vi "DSC Dashboard.vi"() -> ()   [LabVIEW 2016]
uses:
  OAuth/OO OAuth/scope_needed.ctl
  <vilib>/addons/_JKI.lib/REST Client/classes/REST Client/HTTP Header.ctl
  <vilib>/addons/_JKI.lib/REST Client/classes/REST Client/REST Client.lvclass
panel:
  out "Response body":string
  in  "Update Button":bool
  in  "OK":bool
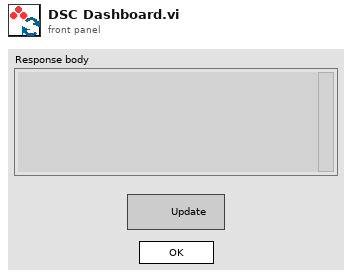
[diagram p1: front panel]
types:
  T1 = enum32{"Invalid", "Standard", "Closed", "Hidden", "Minimized", "Maximized"}
  T2 = enum32{"invalid app kind", "Development System", "Run Time System", "Student Edition", "Embedded LabVIEW", "Evaluation", "Custom"}
  T3 = cluster{"Client ID":string, "Client Secret":string, "Redirect URI":string, "Token Endpoint":string, "Scope":string}
  T4 = typedef "scope_needed.ctl" = enum16{"No", "Yes"}
  T5 = typedef "REST Client.lvlib/REST Client.lvclass/HTTP Header.ctl" = cluster{"header":string, "value":string}
  T6 = cluster{"Core":cluster{"Current VI Reference":refnum<vi>, "Close Panel on Exit?":bool}, "Access Token":string, "Auth Timeout":dbl, "Refresh Token":string, "DSC Data":cluster{"Cyper Temp":dbl, "PPMS1 Temp":dbl, "PPMS1 B-field":dbl, "PPMS2 Temp":dbl, "PPMS2 B-Field":dbl, "PPMS2 He Level":dbl, "THZ1 Temp":dbl, "THZ1 Humidity":dbl, "THZ1 Dew Pt":dbl}}
  T7 = cluster{"Cyper Temp":dbl, "PPMS1 Temp":dbl, "PPMS1 B-field":dbl, "PPMS2 Temp":dbl, "PPMS2 B-Field":dbl, "PPMS2 He Level":dbl, "THZ1 Temp":dbl, "THZ1 Humidity":dbl, "THZ1 Dew Pt":dbl}
  T8 = cluster{"Current VI Reference":refnum<vi>, "Close Panel on Exit?":bool}
  T9 = cluster{"Cypher Temp":dbl, "PPMS1 Temp":dbl, "PPMS1 B-Field":dbl, "PPMS2 Temp":dbl, "PPMS2 B-field":dbl, "PPMS2 He level":dbl, "THZ1 Temp":dbl, "THZ1 Humidity":dbl, "THZ1 Dew Pt":dbl}
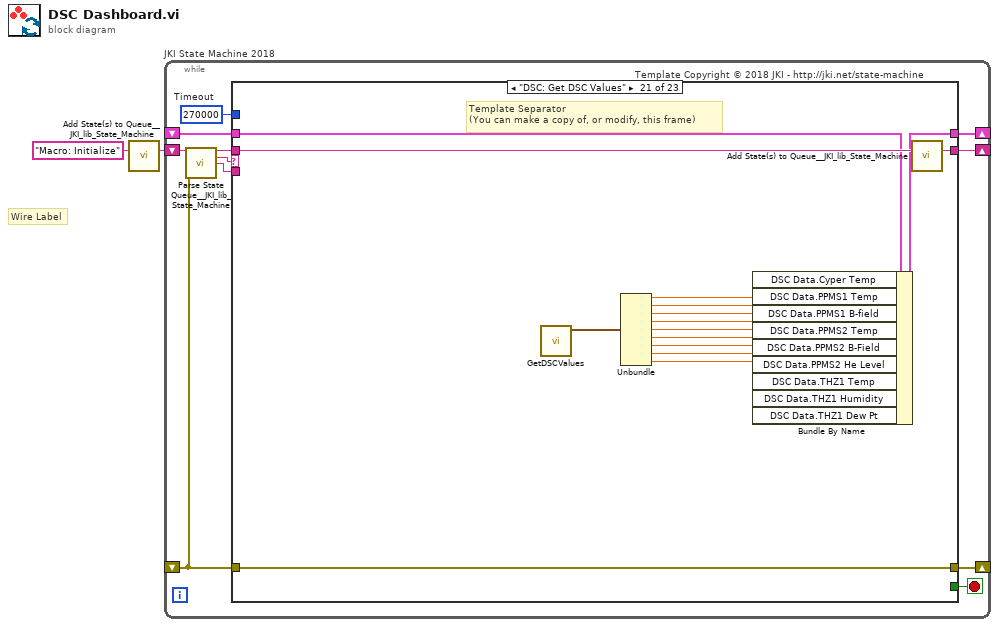
[diagram p0: block diagram]
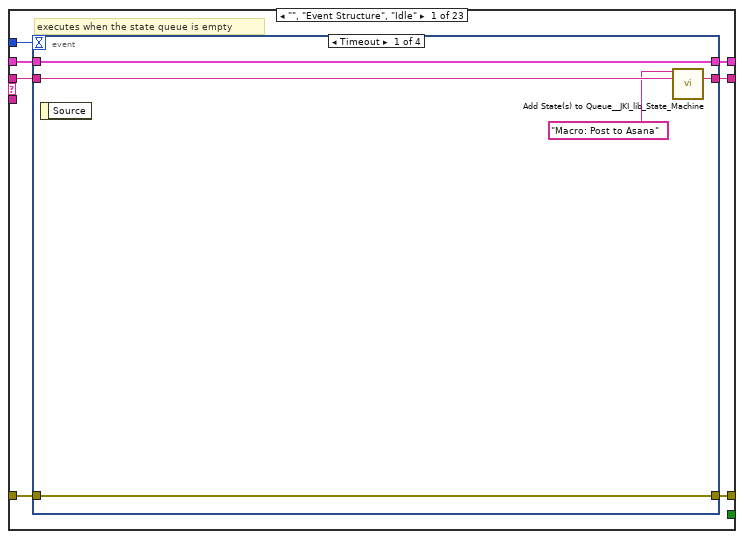
[diagram p2: hidden frame]
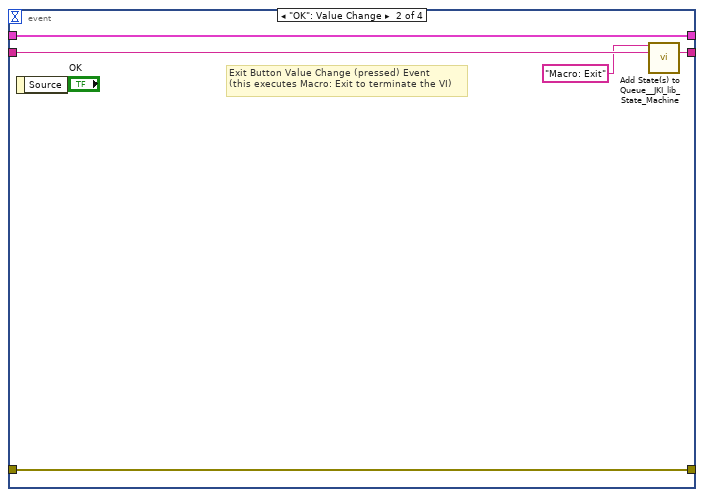
[diagram p3: hidden frame]
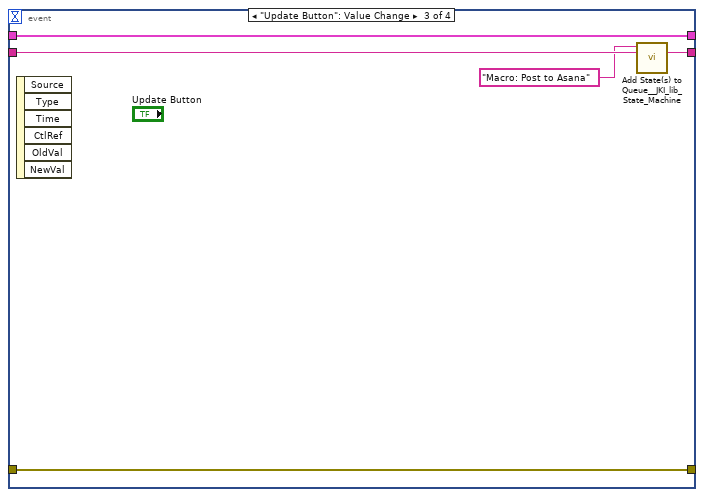
[diagram p4: hidden frame]
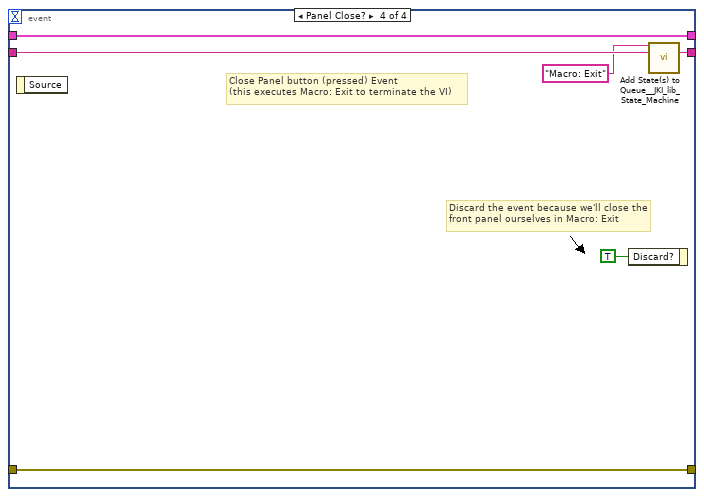
[diagram p5: hidden frame]
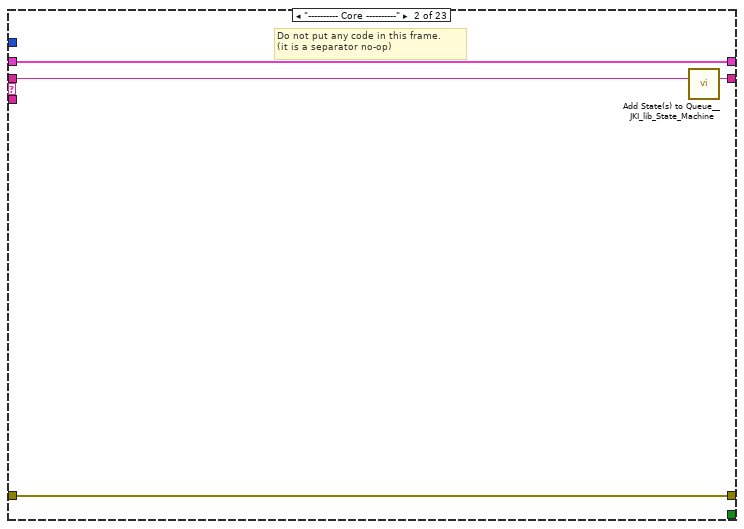
[diagram p6: hidden frame]
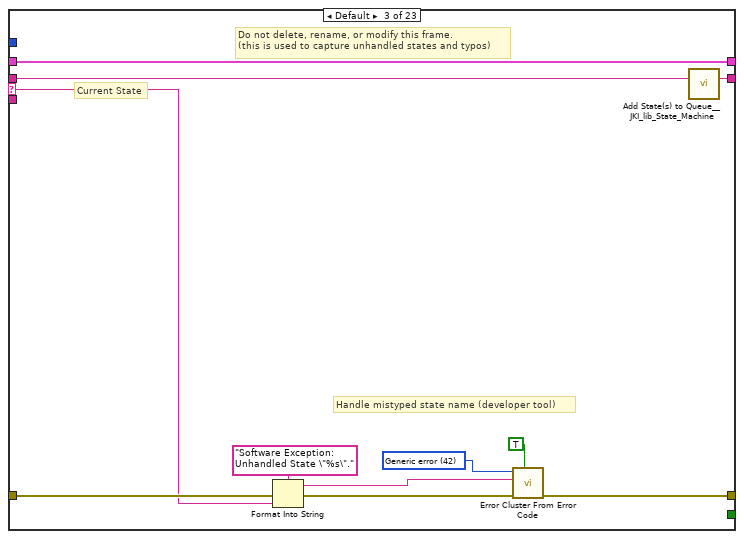
[diagram p7: hidden frame]
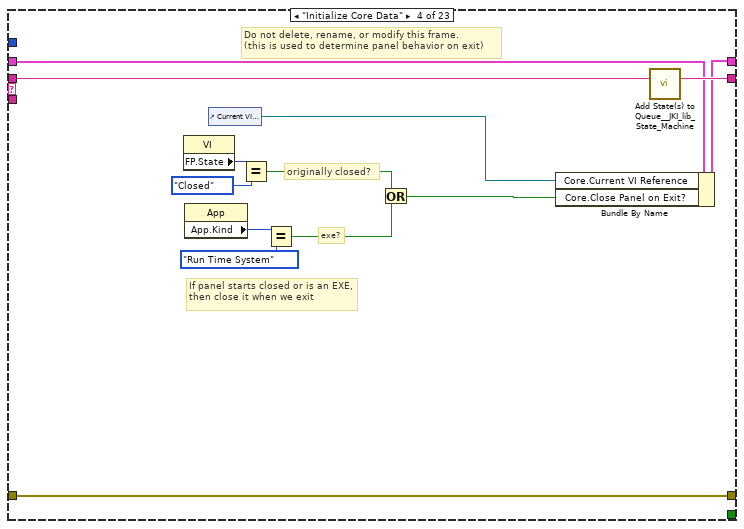
[diagram p8: hidden frame]
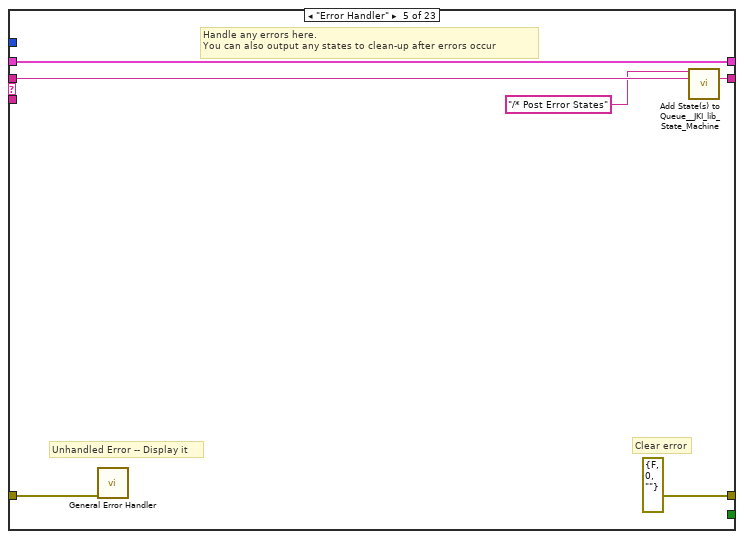
[diagram p9: hidden frame]
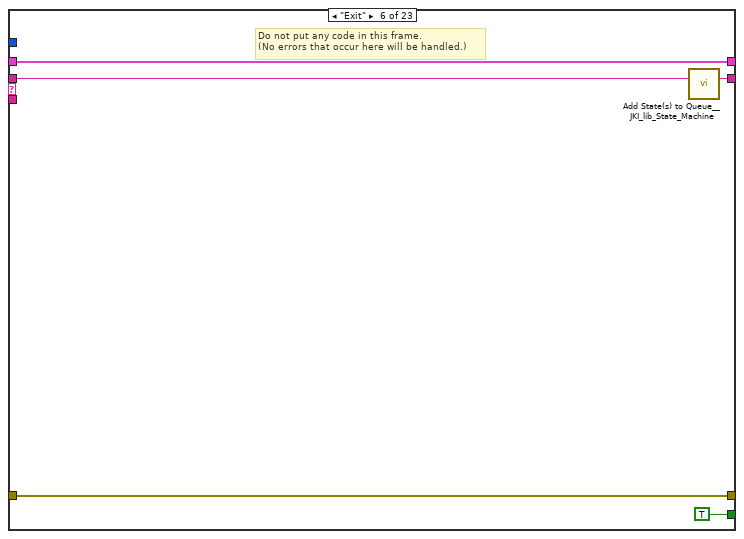
[diagram p10: hidden frame]
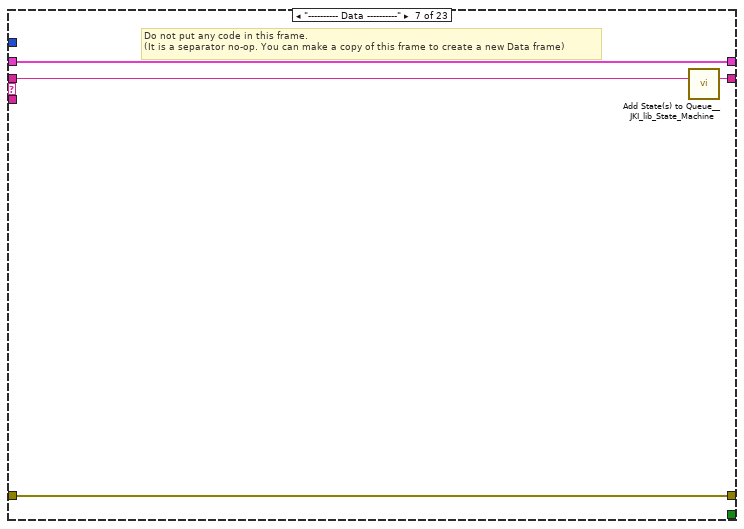
[diagram p11: hidden frame]
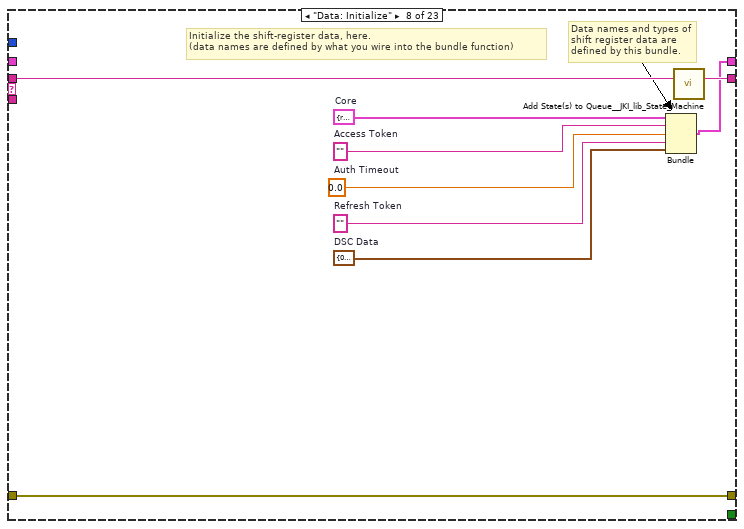
[diagram p12: hidden frame]
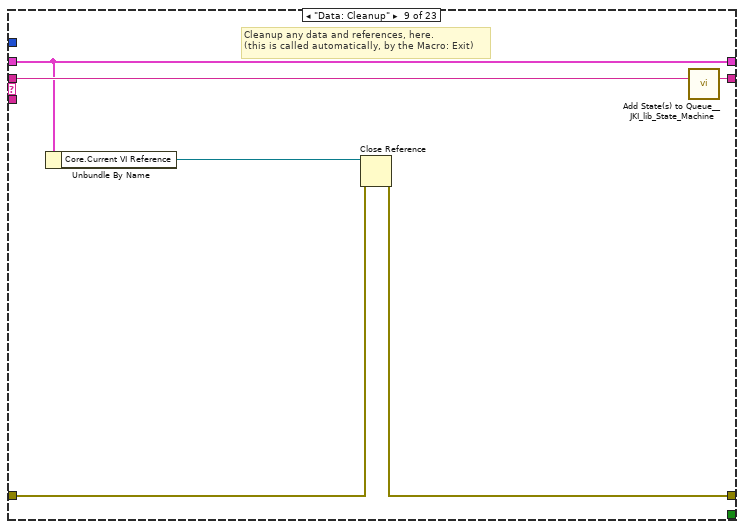
[diagram p13: hidden frame]
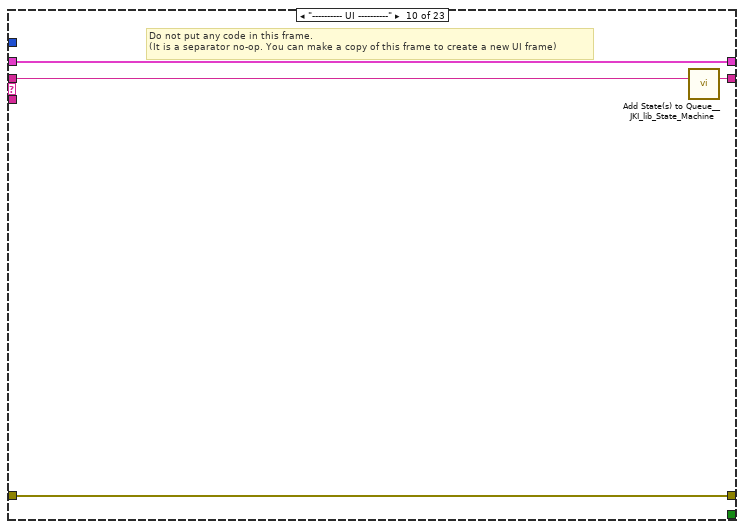
[diagram p14: hidden frame]
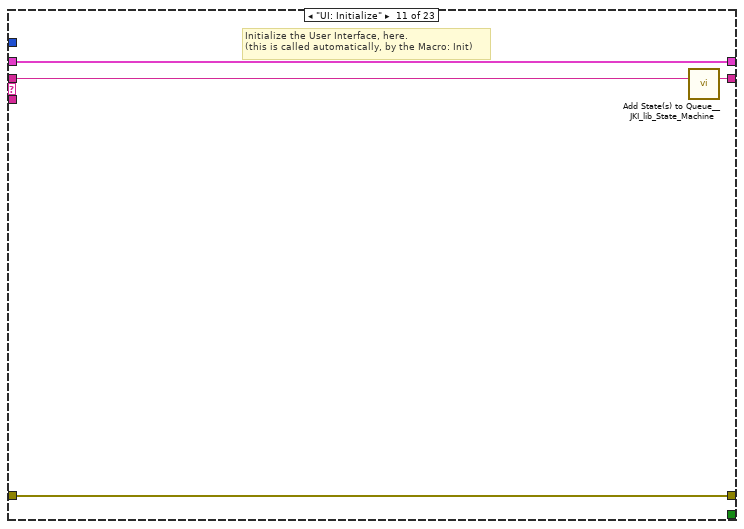
[diagram p15: hidden frame]
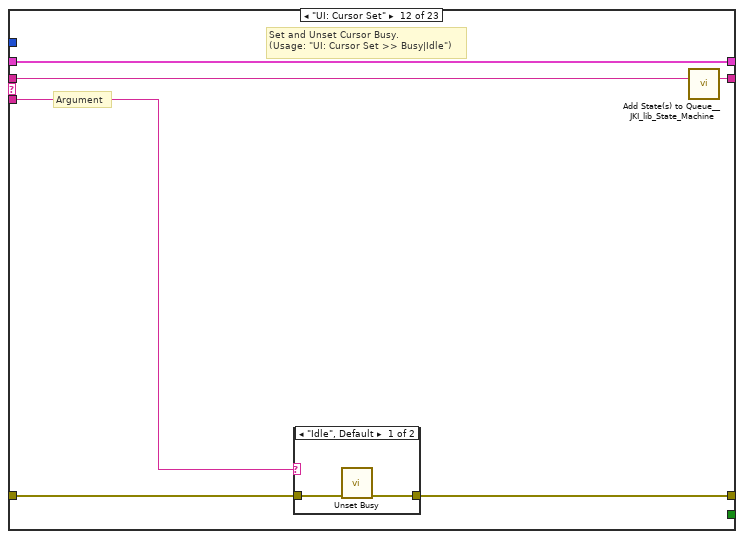
[diagram p16: hidden frame]
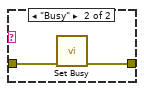
[diagram p17: hidden frame]
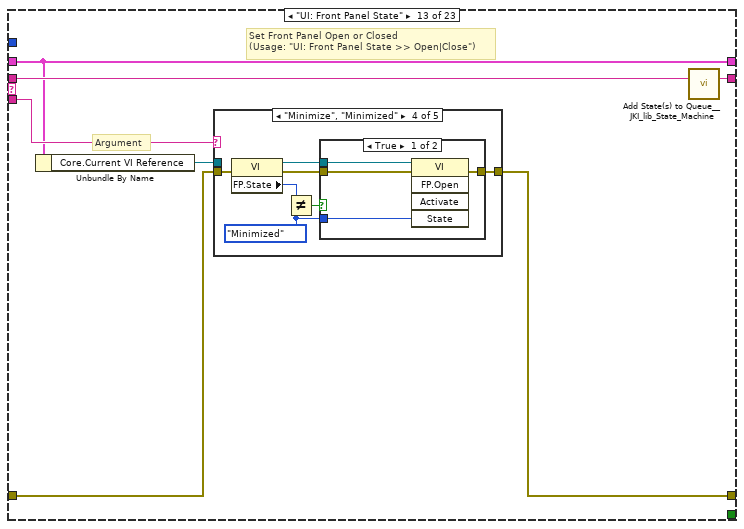
[diagram p18: hidden frame]
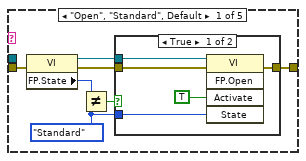
[diagram p19: hidden frame]
diagram:
  # "Wire Label"
  n1 = call <vilib>:"Add State(s) to Queue__JKI_lib_State_Machine.vi"("State(s) in (\"\")"="Macro: Initialize") -> ("States Out"=w2:string)  [unwired: 14 in]
  n2 = while "JKI State Machine 2018" {
    shift-right: [w3] -> _
    shift-left: _ -> [w6]
    shift-right: [w9] -> _
    shift-left: _ -> [w4]
    shift-right: [w8] -> _
    shift-left: w2 -> [w10]
    stop <- w7 stop-if-true
    w5 = 270000  # Timeout
    # "Template Copyright © 2018 JKI - http://jki.net/state-machine"
    n3 = call <vilib>:"Parse State Queue__JKI_lib_State_Machine.vi"("State Queue"=w10, "Error In (no error)"=w4) -> ("Remaining States"=w12:string, "Current State"=w13:string, "Arguments"=w11:string)  [unwired: 11 in]
    n4 = case shown="\"DSC: Get DSC Values\"" w13 {
      selector: w13 -> [_ _ w46 _ _ _ _ _ _ _ _ _ _ _ _ _ _ _ _ _ _ _ _]
      tunnel: w12 -> [w20 w45 w50 w69 w75 w80 w84 w93 w99 w103 w107 w113 w124 w188 w193 w198 w208 w212 w223 w239 w254 w258 w280]
      tunnel: w11 -> [_ _ _ _ _ _ _ _ _ _ _ w108 w119 _ _ _ _ _ _ _ _ _ _]
      tunnel: w6 -> [w18 w42 w48 w57 w72 w78 w81 _ w94 w100 w105 w111 w118 w185 w190 w195 w200 w209 w215 w236 w241 w255 w263]
      tunnel: [w17 w43 w52 w67 errorcluster {"status"=FALSE, "code"=0, "source"=""} ("error out") w77 w82 w91 w96 w101 w104 w109 w121 w186 w191 w196 w206 w210 w216 w237 w252 w256 w259] -> w9
      tunnel: w4 -> [w16 w43 w51 w67 w71 w77 w82 w91 w97 w101 w104 w110 w122 w186 w191 w196 w206 w210 w217 w237 w252 w256 w262]
      tunnel: [w19 w44 w49 w68 w74 w79 w83 w92 w98 w102 w106 w112 w123 w187 w192 w197 w207 w211 w222 w238 w253 w257 w279] -> w8
      tunnel: [_ _ _ _ _ TRUE _ _ _ _ _ _ _ _ _ _ _ _ _ _ _ _ _] -> w7
      tunnel: w5 -> [w14 _ _ _ _ _ _ _ _ _ _ _ _ _ _ _ _ _ _ _ _ _ _]
      tunnel: [w15 w42 w48 w58 w72 w78 w81 w88 w94 w100 w105 w111 w118 w185 w190 w195 w200 w209 w214 w236 w240 w255 w263] -> w3
      frame "", "Event Structure", "Idle" {
        # "executes when the state queue is empty"
        n5 = event shown="[0] Timeout" {
          selector: _ -> [_ _ _ _]
          dyn-events: _ -> [_ _ _ _]
          timeout: w14 -> [_ _ _ _]
          tunnel: w20 -> [w25 w30 w33 w41]
          tunnel: [w24 w29 w34 w40] -> w19
          tunnel: w18 -> [w22 w27 w35 w38]
          tunnel: [w23 w28 w31 w39] -> w17
          tunnel: w16 -> [w23 w28 w31 w39]
          tunnel: [w22 w27 w35 w38] -> w15
          event Timeout {
            n6 = event-data() -> ()  [unwired: 1 in, 1 out]
            n7 = call <vilib>:"Add State(s) to Queue__JKI_lib_State_Machine.vi"("State(s) in Front (\"\")"="Macro: Post to Asana" ("State(s) in Front (\"\")"), "State(s) in (\"\")"=w25) -> ("States Out"=w24:string)  [unwired: 13 in]
          }
          event "OK": Value Change {
            # "Exit Button Value Change (pressed) Event\n(this executes Macro: Exit to terminate the VI)"
            n8 = event-data() -> ()  [unwired: 1 in, 1 out]
            n9 = call <vilib>:"Add State(s) to Queue__JKI_lib_State_Machine.vi"("State(s) in Front (\"\")"="Macro: Exit", "State(s) in (\"\")"=w30) -> ("States Out"=w29:string)  [unwired: 13 in]
          }
          event "Update Button": Value Change {
            n10 = event-data() -> ()  [unwired: 1 in, 6 out]
            n11 = call <vilib>:"Add State(s) to Queue__JKI_lib_State_Machine.vi"("State(s) in Front (\"\")"="Macro: Post to Asana", "State(s) in (\"\")"=w33) -> ("States Out"=w34:string)  [unwired: 13 in]
          }
          event Panel Close? {
            # "Discard the event because we'll close the front panel ourselves in Macro: Exit"
            # "Close Panel button (pressed) Event\n(this executes Macro: Exit to terminate the VI)"
            n12 = event-data() -> ()  [unwired: 1 in, 1 out]
            n13 = event-data("Discard?"=TRUE) -> ()  [unwired: 1 in, 1 out]
            n14 = call <vilib>:"Add State(s) to Queue__JKI_lib_State_Machine.vi"("State(s) in Front (\"\")"="Macro: Exit", "State(s) in (\"\")"=w41) -> ("States Out"=w40:string)  [unwired: 13 in]
          }
        }
      }
      frame "---------- Core ----------" {
        # "Do not put any code in this frame.\n(it is a separator no-op)"
        n15 = call <vilib>:"Add State(s) to Queue__JKI_lib_State_Machine.vi"("State(s) in (\"\")"=w45) -> ("States Out"=w44:string)  [unwired: 14 in]
      }
      frame Default {
        w55 = 42 items=["No error", "Argument error", "Memory is full", "Out of zone", "End of file", "File already open", "Generic file I/O error", "File not found", "File permission error", "Disk is full", "Duplicate path", "Too many files open", "System feature not enabled", "Resource file not found", "Cannot add resource", "Resource not found", "Image not found", "Image memory error", "Pen does not exist", "Config type invalid", "Config token not found", "Config parse error", "Config memory error", "Bad external code format", "Bad external code offset", "External code not present", "Null window", "Destroy window error", "Null menu", "Print aborted", "Bad print record", "Print driver error", "Windows error during printing", "Memory error during printing", "Print dialog error", "Generic print error", "Invalid device refnum", "Device not found", "Device parameter error", "Device unit error", "Cannot open device", "Device call aborted", "Generic error", "Cancelled by user", "Object ID too low", "Object ID too high", "Object not in heap", "Unknown heap", "Unknown object (invalid DefProc)", "Unknown object (DefProc not in table)", "Message out of range", "Invalid (null) method", "Unknown message", "Manager call not supported", "Bad address", "Network operation in progress", "Network operation timed out", "Connection is busy", "Network attribute not supported", "Network error", "Address in use", "System out of memory", "Connection aborted", "Connection refused", "Not connected", "Already connected", "Connection closed", "Initialization error (interapplication manager)", "Bad occurrence", "Wait on unbound occurrence handler", "Occurrence queue overflow", "Datalog type conflict", "Unused", "Unrecognized type (interapplication manager)", "Memory corrupt", "Failed to make temporary DLL", "Old CIN version", "Drag socket not found", "Failed to load drop-object", "Failed to register OLE object", "Failed to release OLE object", "Format specifier type mismatch", "Unknown format specifier", "Too few format specifiers", "Too many format specifiers", "Scan failed", "Newer CIN version", "Error converting to variant", "Runtime menu error", "Password tampered", "Variant attribute not found", "Incompatible variant data type", "Event data is not available", "Event Store is not present", "Occurrence is not found", "Event Queue is not created", "Event info is not available", "Refnum passed is NULL", "Error retrieving Class GUID", "Error retrieving CoClass GUID", "Error retrieving TypeLib GUID.", "Bad built application magic bytes.", "Specific driver is different from the specific driver associated with the Logical Name.", "There is no session opened to the class driver.", "Max Error", "MAX - Error with config objects", "MAX - Error loading configuration", "MAX - Group not supported"]
        # "Current State"
        # "Do not delete, rename, or modify this frame.\n(this is used to capture unhandled states and typos)"
        # "Handle mistyped state name (developer tool)"
        n16 = Format Into String(format string="Software Exception: Unhandled State \"%s\"." ("message"), error in=w51, w46) -> (resulting string=w54:string, error out=w53:errorcluster)  [unwired: 1 in]
        n17 = call <vilib>:"Error Cluster From Error Code.vi"("show call chain? (False)"=TRUE, "error in (no error)"=w53, "error message (\"\")"=w54, "error code (0)"=w55) -> ("error out"=w52:errorcluster)  [unwired: 5 in]
        n18 = call <vilib>:"Add State(s) to Queue__JKI_lib_State_Machine.vi"("State(s) in (\"\")"=w50) -> ("States Out"=w49:string)  [unwired: 14 in]
      }
      frame "Initialize Core Data" {
        # "Do not delete, rename, or modify this frame.\n(this is used to determine panel behavior on exit)"
        # "originally closed?"
        # "exe?"
        # "If panel starts closed or is an EXE, then close it when we exit"
        n19 = property class="VI"() -> ("FP.State"=w61:T1)  [unwired: 2 in, 2 out]
        n20 = property class="App"() -> ("App.Kind"=w66:T2)  [unwired: 2 in, 2 out]
        n21 = control-ref of="Current VI Reference"() -> (w62:refnum<vi>)
        n22 = Equal?(x=w61, y=T1."Closed" ("Front Panel Window:State")) -> (x = y?=w59:bool)
        n23 = Equal?(x=w66, y=T2."Run Time System" ("Application:Kind")) -> (x = y?=w64:bool)
        n24 = Or(x=w59, y=w64) -> (x .or. y?=w63:bool)
        n25 = Bundle By Name(cluster=w57, "Core.Current VI Reference"=w62, "Core.Close Panel on Exit?"=w63) -> (w58:T6)
        n26 = call <vilib>:"Add State(s) to Queue__JKI_lib_State_Machine.vi"("State(s) in (\"\")"=w69) -> ("States Out"=w68:string)  [unwired: 14 in]
      }
      frame "Error Handler" {
        # "Unhandled Error -- Display it"
        # "Handle any errors here.\nYou can also output any states to clean-up after errors occur"
        # "Clear error"
        n27 = call <vilib>:"General Error Handler.vi"("error in (no error)"=w71) -> ()  [unwired: 10 in, 5 out]
        n28 = call <vilib>:"Add State(s) to Queue__JKI_lib_State_Machine.vi"("State(s) in Front (\"\")"="/* Post Error States", "State(s) in (\"\")"=w75) -> ("States Out"=w74:string)  [unwired: 13 in]
      }
      frame "Exit" {
        # "Do not put any code in this frame.\n(No errors that occur here will be handled.)"
        n29 = call <vilib>:"Add State(s) to Queue__JKI_lib_State_Machine.vi"("State(s) in (\"\")"=w80) -> ("States Out"=w79:string)  [unwired: 14 in]
      }
      frame "---------- Data ----------" {
        # "Do not put any code in this frame.\n(It is a separator no-op. You can make a copy of this frame to create a new Data frame)"
        n30 = call <vilib>:"Add State(s) to Queue__JKI_lib_State_Machine.vi"("State(s) in (\"\")"=w84) -> ("States Out"=w83:string)  [unwired: 14 in]
      }
      frame "Data: Initialize" {
        w85 = T7 {"Cyper Temp"=0.0, "PPMS1 Temp"=0.0, "PPMS1 B-field"=0.0, "PPMS2 Temp"=0.0, "PPMS2 B-Field"=0.0, "PPMS2 He Level"=0.0, "THZ1 Temp"=0.0, "THZ1 Humidity"=0.0, "THZ1 Dew Pt"=0.0}  # DSC Data
        w86 = ""  # Refresh Token
        w87 = ""  # Access Token
        w89 = 0.0  # Auth Timeout
        w90 = T8 {"Current VI Reference"=refnum, "Close Panel on Exit?"=FALSE}  # Core
        # "Data names and types of shift register data are defined by this bundle."
        # "Initialize the shift-register data, here.\n(data names are defined by what you wire into the bundle function)"
        n31 = Bundle("Core"=w90, "Access Token"=w87, "Auth Timeout"=w89, "Refresh Token"=w86, "DSC Data"=w85) -> (w88:T6)  [unwired: 1 in]
        n32 = call <vilib>:"Add State(s) to Queue__JKI_lib_State_Machine.vi"("State(s) in (\"\")"=w93) -> ("States Out"=w92:string)  [unwired: 14 in]
      }
      frame "Data: Cleanup" {
        # "Cleanup any data and references, here.\n(this is called automatically, by the Macro: Exit)"
        n33 = Unbundle By Name(w94) -> ("Core.Current VI Reference"=w95:refnum<vi>)
        n34 = Close Reference(reference=w95, error in (no error)=w97) -> (error out=w96:errorcluster)
        n35 = call <vilib>:"Add State(s) to Queue__JKI_lib_State_Machine.vi"("State(s) in (\"\")"=w99) -> ("States Out"=w98:string)  [unwired: 14 in]
      }
      frame "---------- UI ----------" {
        # "Do not put any code in this frame.\n(It is a separator no-op. You can make a copy of this frame to create a new UI frame)"
        n36 = call <vilib>:"Add State(s) to Queue__JKI_lib_State_Machine.vi"("State(s) in (\"\")"=w103) -> ("States Out"=w102:string)  [unwired: 14 in]
      }
      frame "UI: Initialize" {
        # "Initialize the User Interface, here.\n(this is called automatically, by the Macro: Init)"
        n37 = call <vilib>:"Add State(s) to Queue__JKI_lib_State_Machine.vi"("State(s) in (\"\")"=w107) -> ("States Out"=w106:string)  [unwired: 14 in]
      }
      frame "UI: Cursor Set" {
        # "Argument"
        # "Set and Unset Cursor Busy.\n(Usage: \"UI: Cursor Set >> Busy|Idle\")"
        n38 = case shown="\"Idle\", Default" w108 {
          tunnel: w110 -> [w115 w117]
          tunnel: [w114 w116] -> w109
          frame "Idle", Default {
            n39 = call <vilib>:"Unset Busy.vi"("error in (no error)"=w115) -> ("error out"=w114:errorcluster)  [unwired: 10 in]
          }
          frame "Busy" {
            n40 = call <vilib>:"Set Busy.vi"("error in (no error)"=w117) -> ("error out"=w116:errorcluster)  [unwired: 9 in, 1 out]
          }
        }
        n41 = call <vilib>:"Add State(s) to Queue__JKI_lib_State_Machine.vi"("State(s) in (\"\")"=w113) -> ("States Out"=w112:string)  [unwired: 14 in]
      }
      frame "UI: Front Panel State" {
        # "Argument"
        # "Set Front Panel Open or Closed\n(Usage: \"UI: Front Panel State >> Open|Close\")"
        n42 = Unbundle By Name(w118) -> ("Core.Current VI Reference"=w120:refnum<vi>)
        n43 = case shown="\"Minimize\", \"Minimized\"" w119 {
          tunnel: w122 -> [w130 w143 w154 w166 w178]
          tunnel: [w131 w144 w155 w167 w179] -> w121
          tunnel: w120 -> [_ _ _ _ _]
          frame "Open", "Standard", Default {
            w125 = T1."Standard" ("State")
            n44 = property class="VI"(error in=w130) -> (reference out=w128:refnum<vi>, error out=w129:errorcluster, "FP.State"=w127:T1)  [unwired: 1 in]
            n45 = Not Equal?(x=w127, y=w125) -> (x != y?=w126:bool)
            n46 = case shown="True" w126 {
              tunnel: [w135 w137] -> w131
              tunnel: w129 -> [w134 w137]
              tunnel: w128 -> [w133 _]
              tunnel: w125 -> [w132 _]
              frame True {
                n47 = invoke class="VI" method="FP.Open"(reference=w133, error in=w134, "Activate"=TRUE, "State"=w132) -> (error out=w135:errorcluster)  [unwired: 1 in, 4 out]
              }
              frame False {
              }
            }
          }
          frame "Close", "Closed" {
            n48 = property class="VI"(error in=w143) -> (reference out=w141:refnum<vi>, error out=w142:errorcluster, "FP.State"=w139:T1)  [unwired: 1 in]
            n49 = Not Equal?(x=w139, y=T1."Closed" ("Front Panel Window:State")) -> (x != y?=w138:bool)
            n50 = case shown="True" w138 {
              tunnel: [w145 w148] -> w144
              tunnel: w142 -> [w145 w147]
              tunnel: w141 -> [_ w146]
              frame False {
              }
              frame True {
                n51 = invoke class="VI" method="FP.Close"(reference=w146, error in=w147) -> (error out=w148:errorcluster)  [unwired: 1 in, 2 out]
              }
            }
          }
          frame "Hidden", "Hide" {
            w149 = T1."Hidden" ("State")
            n52 = property class="VI"(error in=w154) -> (reference out=w152:refnum<vi>, error out=w153:errorcluster, "FP.State"=w151:T1)  [unwired: 1 in]
            n53 = Not Equal?(x=w151, y=w149) -> (x != y?=w150:bool)
            n54 = case shown="True" w150 {
              tunnel: [w159 w160] -> w155
              tunnel: w153 -> [w158 w160]
              tunnel: w152 -> [w157 _]
              tunnel: w149 -> [w156 _]
              frame True {
                n55 = invoke class="VI" method="FP.Open"(reference=w157, error in=w158, "State"=w156) -> (error out=w159:errorcluster)  [unwired: 2 in, 4 out]
              }
              frame False {
              }
            }
          }
          frame "Minimize", "Minimized" {
            w161 = T1."Minimized" ("State")
            n56 = property class="VI"(error in=w166) -> (reference out=w164:refnum<vi>, error out=w165:errorcluster, "FP.State"=w163:T1)  [unwired: 1 in]
            n57 = Not Equal?(x=w163, y=w161) -> (x != y?=w162:bool)
            n58 = case shown="True" w162 {
              tunnel: [w171 w172] -> w167
              tunnel: w165 -> [w170 w172]
              tunnel: w164 -> [w169 _]
              tunnel: w161 -> [w168 _]
              frame True {
                n59 = invoke class="VI" method="FP.Open"(reference=w169, error in=w170, "State"=w168) -> (error out=w171:errorcluster)  [unwired: 2 in, 4 out]
              }
              frame False {
              }
            }
          }
          frame "Maximize", "Maximized" {
            w173 = T1."Maximized" ("State")
            n60 = property class="VI"(error in=w178) -> (reference out=w176:refnum<vi>, error out=w177:errorcluster, "FP.State"=w175:T1)  [unwired: 1 in]
            n61 = Not Equal?(x=w175, y=w173) -> (x != y?=w174:bool)
            n62 = case shown="True" w174 {
              tunnel: [w183 w184] -> w179
              tunnel: w177 -> [w182 w184]
              tunnel: w176 -> [w181 _]
              tunnel: w173 -> [w180 _]
              frame True {
                n63 = invoke class="VI" method="FP.Open"(reference=w181, error in=w182, "State"=w180) -> (error out=w183:errorcluster)  [unwired: 2 in, 4 out]
              }
              frame False {
              }
            }
          }
        }
        n64 = call <vilib>:"Add State(s) to Queue__JKI_lib_State_Machine.vi"("State(s) in (\"\")"=w124) -> ("States Out"=w123:string)  [unwired: 14 in]
      }
      frame "---------- Macro ----------" {
        # "Do not put any code in this frame.\n(It is a separator no-op. You can make a copy of this frame to create a new Macro frame)"
        n65 = call <vilib>:"Add State(s) to Queue__JKI_lib_State_Machine.vi"("State(s) in (\"\")"=w188) -> ("States Out"=w187:string)  [unwired: 14 in]
      }
      frame "Macro: Post to Asana" {
        # "Do not put any code in this frame.\n(It is a separator no-op. You can make a copy of this frame to create a new Macro frame)"
        n66 = call <vilib>:"Add State(s) to Queue__JKI_lib_State_Machine.vi"("State(s) in Front (\"\")"="Authorization: Handle\nDSC: Get DSC Values\nAsana: Post to Asana" ("State(s) in Front (\"\")"), "State(s) in (\"\")"=w193) -> ("States Out"=w192:string)  [unwired: 13 in]
      }
      frame "Macro: Initialize" {
        w194 = "Data: Initialize\nInitialize Core Data\nUI: Initialize\nUI: Front Panel State >> Open"  # Data: Initialize Initialize Core Data UI: Initialize UI: Front Panel State >> Open
        # "Initialization Macro\n(This is called once, when the VI starts)"
        n67 = call <vilib>:"Add State(s) to Queue__JKI_lib_State_Machine.vi"("State(s) in Front (\"\")"=w194, "State(s) in (\"\")"=w198) -> ("States Out"=w197:string)  [unwired: 13 in]
      }
      frame "Macro: Exit" {
        # "Exit Macro\n(This is called once, when the VI exits)"
        n68 = Unbundle By Name(w200) -> ("Core.Close Panel on Exit?"=w199:bool)
        n69 = Select(t="UI: Front Panel State >> Close", s=w199, f="") -> (s? t:f=w203:string)
        n70 = call <vilib>:"Add State(s) to Queue__JKI_lib_State_Machine.vi"("State(s) in (\"\")"=w203, "State(s) at Back (\"\")"="Data: Cleanup\nExit") -> ("States Out"=w201:string)  [unwired: 13 in]
        n71 = call <vilib>:"Add State(s) to Queue__JKI_lib_State_Machine.vi"("State(s) in Front (\"\")"=w201, "State(s) in (\"\")"=w208) -> ("States Out"=w207:string)  [unwired: 13 in]
      }
      frame "---------- Authorization ----------" {
        # "Template Separator\n(You can make a copy of, or modify, this frame)"
        n72 = call <vilib>:"Add State(s) to Queue__JKI_lib_State_Machine.vi"("State(s) in (\"\")"=w212) -> ("States Out"=w211:string)  [unwired: 14 in]
      }
      frame "Authorization: Handle" {
        # "If it is, reauthenticate.\nIf not, do nothing."
        # "Check if the current time is\ngreater than the authentication\ndeadline"
        n73 = Get Date/Time In Seconds() -> (seconds since 1Jan1904=w221:timestamp)
        n74 = Unbundle By Name(w215) -> ("Auth Timeout"=w220:dbl, "Refresh Token"=w213:string)
        n75 = To Double Precision Float(number=w221) -> (double precision float=w218:dbl)
        n76 = Less Or Equal?(x=w220, y=w218) -> (x <= y?=w219:bool)
        n77 = case shown="True" w219 {
          tunnel: w217 -> [w225 w233]
          tunnel: [w225 w232] -> w216
          tunnel: w215 -> [w224 w231]
          tunnel: [w224 w230] -> w214
          tunnel: w213 -> [_ w227]
          frame False {
          }
          frame True {
            n78 = call "Authenticate.vi"("error in (no error)"=w233, "Refresh Token"=w227, "Authentication Info"=T3 {"Client ID"="1108428692000476", "Client Secret"="803bdca1138fccb00921b8f346728904", "Redirect URI"="https://app.asana.com/api/1.0", "Token Endpoint"="https://app.asana.com/-/oauth_token", "Scope"=""}, "Scope Needed?"=scope_needed."No") -> ("error out"=w232:errorcluster, "Refresh Token"=w226:string, "Timeout"=w234:dbl, "Access Token"=w235:string)  [unwired: 4 in]
            n79 = Bundle By Name(cluster=w231, "Access Token"=w235, "Auth Timeout"=w234, "Refresh Token"=w226) -> (w230:T6)
          }
        }
        n80 = call <vilib>:"Add State(s) to Queue__JKI_lib_State_Machine.vi"("State(s) in (\"\")"=w223) -> ("States Out"=w222:string)  [unwired: 14 in]
      }
      frame "---------- DSC ----------" {
        # "Template Separator\n(You can make a copy of, or modify, this frame)"
        n81 = call <vilib>:"Add State(s) to Queue__JKI_lib_State_Machine.vi"("State(s) in (\"\")"=w239) -> ("States Out"=w238:string)  [unwired: 14 in]
      }
      frame "DSC: Get DSC Values" {
        # "Template Separator\n(You can make a copy of, or modify, this frame)"
        n82 = call "GetDSCValues.vi"() -> ("cluster"=w251:T9)  [unwired: 11 in]
        n83 = Unbundle(w251) -> ("Cypher Temp"=w250:dbl, "PPMS1 Temp"=w249:dbl, "PPMS1 B-Field"=w248:dbl, "PPMS2 Temp"=w247:dbl, "PPMS2 B-field"=w246:dbl, "PPMS2 He level"=w244:dbl, "THZ1 Temp"=w245:dbl, "THZ1 Humidity"=w243:dbl, "THZ1 Dew Pt"=w242:dbl)
        n84 = Bundle By Name(cluster=w241, "DSC Data.Cyper Temp"=w250, "DSC Data.PPMS1 Temp"=w249, "DSC Data.PPMS1 B-field"=w248, "DSC Data.PPMS2 Temp"=w247, "DSC Data.PPMS2 B-Field"=w246, "DSC Data.PPMS2 He Level"=w244, "DSC Data.THZ1 Temp"=w245, "DSC Data.THZ1 Humidity"=w243, "DSC Data.THZ1 Dew Pt"=w242) -> (w240:T6)
        n85 = call <vilib>:"Add State(s) to Queue__JKI_lib_State_Machine.vi"("State(s) in (\"\")"=w254) -> ("States Out"=w253:string)  [unwired: 14 in]
      }
      frame "---------- Asana ----------" {
        # "Template Separator\n(You can make a copy of, or modify, this frame)"
        n86 = call <vilib>:"Add State(s) to Queue__JKI_lib_State_Machine.vi"("State(s) in (\"\")"=w258) -> ("States Out"=w257:string)  [unwired: 14 in]
      }
      frame "Asana: Post to Asana" {
        # "Template Separator\n(You can make a copy of, or modify, this frame)"
        n87 = Unbundle By Name(w263) -> ("Access Token"=w269:string)
        n88 = Concatenate Strings("Bearer ", w269) -> (w268:string)
        n89 = Bundle By Name(cluster=T5 {"header"="", "value"=""} ("Header"), "header"="Authorization", "value"=w268) -> (w266:T5)
        n90 = call <vilib>:"Create REST Client.vi"("error in (no error)"=w262, "Base URL"="https://app.asana.com/api/1.0") -> ("error out"=w261:errorcluster, "REST Client out"=w278:refnum<class "REST Client.lvclass">)  [unwired: 8 in]
        n91 = Replace Array Subset(array=T5[] [{"header"="", "value"=""}] ("request specific headers"), new element=w266, index=0) -> (w272:T5[])
        n92 = call-dynamic "HTTP POST.vi"("request specific headers"=w272, "error in (no error)"=w261, "Request body"="{\"data\": {\"projects\": [1123044036758048], \"name\": \"Wow! It's a time knife\", \"notes\": \"https://swordscomic.com/swords/CLXXVIII/\"}}", "Path"="/tasks", "REST Client in"=w278) -> ("error out"=w260:errorcluster, "Response body"=→"Response body":string, "REST Client out"=w277:refnum<class "REST Client.lvclass">)  [unwired: 1 in, 3 out]
        n93 = call-dynamic "Destroy REST Client.vi"("error in (no error)"=w260, "REST Client in"=w277) -> ("error out"=w259:errorcluster)  [unwired: 9 in]
        n94 = call <vilib>:"Add State(s) to Queue__JKI_lib_State_Machine.vi"("State(s) in (\"\")"=w280) -> ("States Out"=w279:string)  [unwired: 14 in]
      }
    }
  }
